vi "Read MsgSerializer.vi"(11 "Test Report in":refnum<class "Test Report.lvclass">) -> (2 "MsgSerializer":refnum<class "MsgSerializer.lvclass">, 3 "Test Report out":refnum<class "Test Report.lvclass">)   [LabVIEW 2020, in "Caraya.lvlib" / "Test Report.lvclass"]
uses:
  Test Report.lvclass
  MsgSerializer/MsgSerializer.lvclass
  Test Report.lvclass/Test Report.ctl
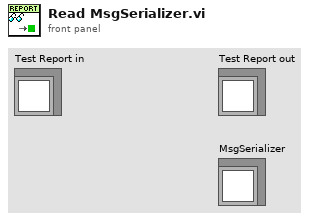
[diagram p1: front panel]
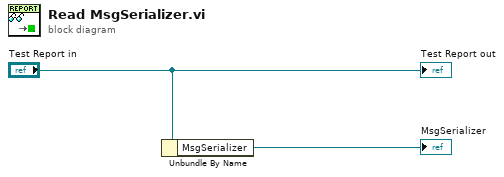
[diagram p0: block diagram]
diagram:
  n1 = Unbundle By Name("Test Report in") -> ("MsgSerializer"=→"MsgSerializer":refnum<class "MsgSerializer.lvclass">)
  "Test Report out" <- "Test Report in"
